vi "DeviceOn.vi"(8 "error in (no error)":errorcluster, 11 "NhRegenGridSim in":refnum<class "NHRGridSim.lvclass">) -> (0 "error out":errorcluster, 3 "NhRegenGridSim out":refnum<class "NHRGridSim.lvclass">)   [LabVIEW 2018, in "AcPwrPlugins.lvlib" / "NHRGridSim.lvclass"]
doc: "This VI (if the unit is not already on) turns on the unit. On is defined as the output relay closed with the unit at zero volts."
uses:
  NHRGridSim.lvclass
  <instrlib>/NH Research 9400 Series/NH Research 9400 Series.lvlib
  <instrlib>/NH Research 9400 Series/Public/Configure/Configure Setpoint (Current).vi
  <instrlib>/NH Research 9400 Series/Public/Configure/Configure Setpoint (Power).vi
  <instrlib>/NH Research 9400 Series/Public/Configure/Configure Setpoint (Voltage).vi
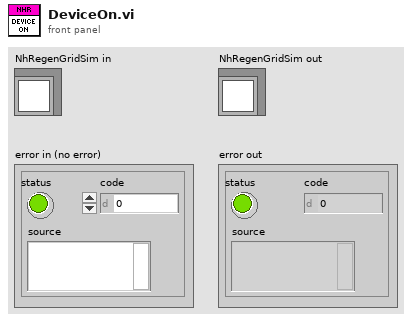
[diagram p1: front panel]
types:
  T1 = typedef "AcPwrPlugins.lvlib/NHRGridSim.lvclass/Device(s)Settings.ctl" = cluster{"MeasName":string, "Instr1":T2, "Instr2":T2, "Instr3":T2, "Handle":string, "Reset":bool, "Mode":T9, "ID Query":bool, "Connected":bool}
  T2 = typedef "AcPwrPlugins.lvlib/NHRGridSim.lvclass/NHRGrid_InstrumentCluster_Tabs.ctl" = cluster{"Name":string, "Vout (V)":dbl, "VType":string, "Phases":T3, "FreqOut (Hz)":dbl, "Aperture (cycles)":i32, "Configure Instrument":T4, "AC Wave Shape":T5, "Ranges":T6, "Safety Trips":T7, "Slew Rates":T8}
  T3 = typedef "AcPwrPlugins.lvlib/NHRGridSim.lvclass/NHRGrid_Phases_Tabs.ctl" = cluster{"A-Volts (V)":dbl, "B-Volts (V)":dbl, "C-Volts (V)":dbl, "Change at (Deg)":i32, "B-Angle (Deg)":i32, "C-Angle (Deg)":i32}
  T4 = typedef "AcPwrPlugins.lvlib/NHRGridSim.lvclass/NHRGrid_Configure_Tabs.ctl" = u16
  T5 = typedef "AcPwrPlugins.lvlib/NHRGridSim.lvclass/NHRGrid_WaveShape_Tabs.ctl" = u16
  T6 = typedef "AcPwrPlugins.lvlib/NHRGridSim.lvclass/NHRGrid_Ranges_Tabs.ctl" = cluster{"Voltage (V)":u16, "Current (A)":u16}
  T7 = typedef "AcPwrPlugins.lvlib/NHRGridSim.lvclass/NHRGrid_SafetyTrips_Tabs.ctl" = cluster{"Vmax (V)":dbl, "Vmin (V)":dbl, "Vmax Time (s)":dbl, "Vmin Time (s)":dbl, "Imax Source (A)":dbl, "Imax Sink (A)":dbl, "I Src Time (s)":dbl, "I Snk Time (s)":dbl, "Pmax Source (W)":dbl, "Pmax Sink (W)":dbl, "P Src Time (s)":dbl, "P Snk Time (s)":dbl, "Abs Volt Peak":dbl, "Enable Vpk":bool, "Abs Curr Peak":dbl, "Enable Ipk":bool}
  T8 = typedef "AcPwrPlugins.lvlib/NHRGridSim.lvclass/NHRGrid_SlewRates_Tabs.ctl" = cluster{"Voltage (V/s)":dbl, "Current (A/s)":dbl, "Power (W/s)":dbl, "Frequency (Hz/s)":dbl, "Phase Angle (Deg/s)":dbl}
  T9 = typedef "AcPwrPlugins.lvlib/NHRGridSim.lvclass/NHRGrid_Modes.ctl" = u8
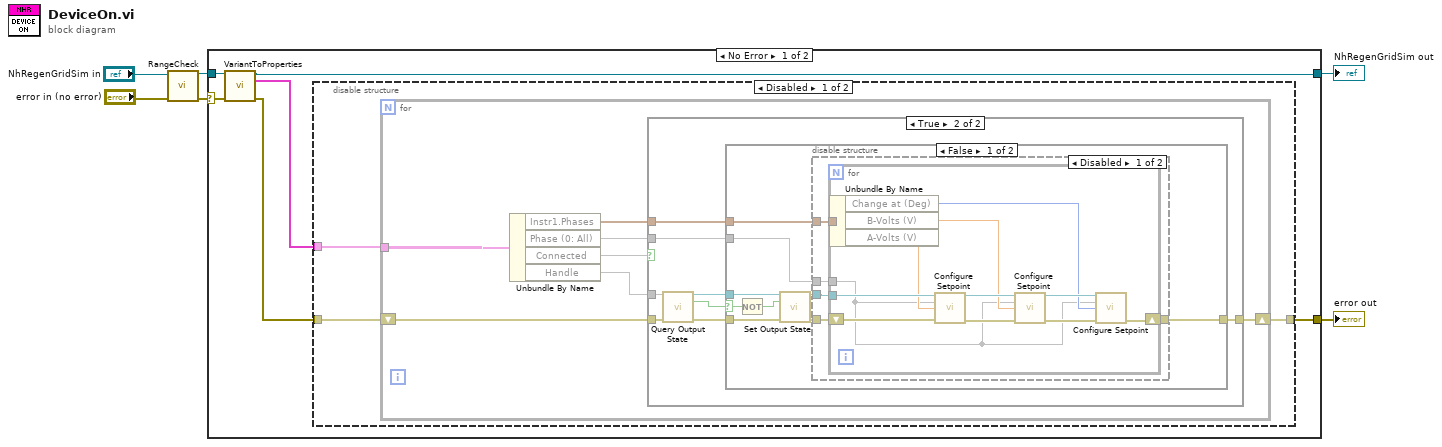
[diagram p0: block diagram]
diagram:
  n1 = call-dynamic "RangeCheck.vi"("NhRegenGridSim in"="NhRegenGridSim in", "error in (no error)"="error in (no error)") -> ("NhRegenGridSim out"=w1:refnum<class "NHRGridSim.lvclass">, "error out"=w3:errorcluster)  [unwired: 7 in]
  n2 = case shown="No Error" w3 {
    selector: w3 -> [w10 w61]
    tunnel: w1 -> [w11 w62]
    tunnel: [w9 w62] -> w6
    tunnel: [w12 w61] -> w5
    frame No Error {
      n3 = call "VariantToProperties.vi"("NHRGridSim in"=w11, "error in (no error)"=w10) -> ("NHRGridSim out"=w9:refnum<class "NHRGridSim.lvclass">, "Device(s)Settings"=w7:T1, "error out"=w8:errorcluster)  [unwired: 8 in, 3 out]
      n4 = disable-structure shown="Disabled" {
        disable-tunnel: [w15 w60] -> w12
        disable-tunnel: w8 -> [w14 w60]
        disable-tunnel: w7 -> [w13 _]
        frame Disabled {
          n5 = for {
            tunnel: w13 -> [w22]
            shift-right: [w20] -> w15
            shift-left: w14 -> [w21]
            n6 = Unbundle By Name(w22) -> ("Instr1.Phases"=w16:T3, "Phase (0: All)"=w17, "Connected"=w18, "Handle"=w19)
            n7 = case shown="True" w18 {
              tunnel: w21 -> [w23 w31]
              tunnel: [w23 w28] -> w20
              tunnel: w19 -> [_ w27]
              tunnel: w17 -> [_ w24]
              tunnel: w16 -> [_ w25]
              frame False {
              }
              frame True {
                n8 = call <instrlib>:"Query Output State.vi"("VISA resource name"=w27, "error in (no error)"=w31) -> ("VISA resource name out"=w26:refnum<visa-resource-name>, "Output Enabled"=w30:bool, "error out"=w29:errorcluster)  [unwired: 11 in]
                n9 = case shown="False" w30 {
                  selector: w30 -> [w38 _]
                  tunnel: w29 -> [w40 w59]
                  tunnel: [w35 w59] -> w28
                  tunnel: w26 -> [w39 _]
                  tunnel: w25 -> [w34 _]
                  tunnel: w24 -> [w33 _]
                  frame False {
                    n10 = Not(x=w38) -> (.not. x?=w37:bool)
                    n11 = call <instrlib>:"Set Output State.vi"("VISA resource name"=w39, "Output State (F: Disable)"=w37, "error in (no error)"=w40) -> ("VISA resource name out"=w32:refnum<visa-resource-name>, "error out"=w36:errorcluster)  [unwired: 11 in]
                    n12 = disable-structure shown="Disabled" {
                      disable-tunnel: w36 -> [w45 w58]
                      disable-tunnel: [w44 w58] -> w35
                      disable-tunnel: w34 -> [w43 _]
                      disable-tunnel: w33 -> [w42 _]
                      disable-tunnel: w32 -> [w41 _]
                      frame Disabled {
                        n13 = for {
                          tunnel: w41 -> [w53]
                          shift-right: [w47] -> w44
                          shift-left: w45 -> [w52]
                          tunnel: w43 -> [w51]
                          tunnel: w42 -> [w46]
                          n14 = Unbundle By Name(w51) -> ("Change at (Deg)"=w48:i32, "B-Volts (V)"=w49:dbl, "A-Volts (V)"=w50:dbl)
                          n15 = call-poly <instrlib>:"Configure Setpoint.vi"("VISA resource name"=w53, "Phase (0: All)"=w46, "Output Power (0 W)"=w50, "error in (no error)"=w52) -> ("VISA resource name out"=w54:refnum<visa-resource-name>, "error out"=w57:errorcluster)  [unwired: 10 in]
                          n16 = call-poly <instrlib>:"Configure Setpoint.vi"("VISA resource name"=w54, "Phase (0: All)"=w46, "Output Current (0 A)"=w49, "error in (no error)"=w57) -> ("VISA resource name out"=w55:refnum<visa-resource-name>, "error out"=w56:errorcluster)  [unwired: 10 in]
                          n17 = call-poly <instrlib>:"Configure Setpoint.vi"("VISA resource name"=w55, "Phase (0: All)"=w46, "Output Voltage (0 V)"=w48, "error in (no error)"=w56) -> ("error out"=w47:errorcluster)  [unwired: 10 in, 1 out]
                        }
                      }
                      frame Enabled {
                      }
                    }
                  }
                  frame True {
                  }
                }
              }
            }
          }
        }
        frame Enabled {
        }
      }
    }
    frame Error {
    }
  }
  "error out" <- w5
  "NhRegenGridSim out" <- w6
